vi "Compute Result.vi"(8 "Y":dbl format="%.5f", 9 "X":dbl format="%.5f", 10 "Full Scale":dbl format="%.5f", 11 "Mode (2: X)":u16(ring)=2 items=["R [V]", "Theta", "X", "Y"]) -> (2 "Computed Value":dbl format="%.2f")   [LabVIEW 2010, in "Stanford Research 844.lvlib"]
doc: "This VI produces X,Y,R or phase."
uses:
  <instrlib>/Stanford Research 844/Stanford Research 844.lvlib
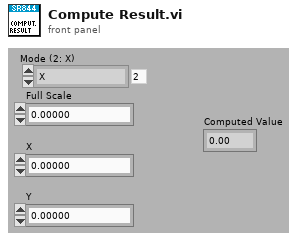
[diagram p1: front panel]
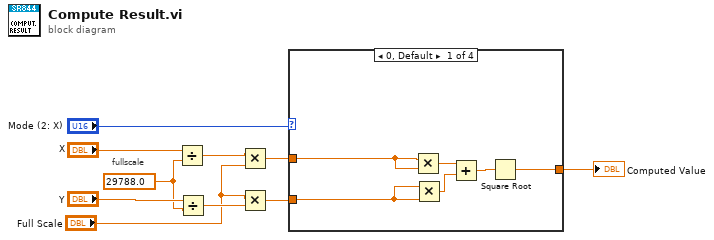
[diagram p0: block diagram]
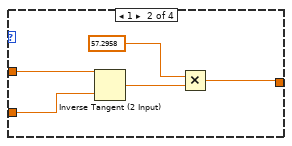
[diagram p2: hidden frame]
diagram:
  w6 = 29788.0 ("y")
  # "fullscale"
  n1 = Divide(x="X", y=w6) -> (x/y=w5:dbl)
  n2 = Divide(x="Y", y=w6) -> (x/y=w2:dbl)
  n3 = Multiply(x=w5, y="Full Scale") -> (x*y=w4:dbl)
  n4 = Multiply(x="Full Scale", y=w2) -> (x*y=w3:dbl)
  n5 = case shown="0, Default" "Mode (2: X)" {
    tunnel: w4 -> [w16 w21 w22 _]
    tunnel: w3 -> [w12 w20 _ w23]
    tunnel: [w14 w17 w22 w23] -> w9
    frame 0, Default {
      n6 = Multiply(x=w16, y=w16) -> (x*y=w13:dbl)
      n7 = Multiply(x=w12, y=w12) -> (x*y=w11:dbl)
      n8 = Add(x=w13, y=w11) -> (x+y=w15:dbl)
      n9 = Square Root(x=w15) -> (sqrt(x)=w14:dbl)
    }
    frame 1 {
      n10 = Inverse Tangent (2 Input)(1:w20, 2:w21) -> (0:w18:dbl)
      n11 = Multiply(x=57.2958, y=w18) -> (x*y=w17:dbl)
    }
    frame 2 {
    }
    frame 3 {
    }
  }
  "Computed Value" <- w9
